vi "Drive_Notifier_Begin.vi"   [LabVIEW 2020]
uses:
  Subsystems/Drive/Drive_Cluster.ctl
  Subsystems/Drive/Drive_Control_States.ctl
  Subsystems/Drive/Drive_Orientation_States.ctl
  Globals/Drive_Globals.vi
types:
  T1 = typedef "Drive_Cluster.ctl" = cluster{"Control_State":T2, "Vertical_Throttle":dbl, "Lateral_Throttle":dbl, "Rotational_Throttle":dbl, "Strafe_In_Deadband":bool, "Rotation_In_Deadband":bool, "Orientation_State":T3, "Parameters":dbl[], "Step":i32, "Auto_Notifier":refnum<notifier>, "PathName":string, "Raw_X":dbl, "Raw_Y":dbl, "Pivot_Driving?":bool}
  T2 = typedef "Drive_Control_States.ctl" = enum16{"No-Op", "Manual_Control", "Command_DriveDistanceAtAngle", "Command_DrivePath", "Command_SetRobotPose", "Command_Rotate"}
  T3 = typedef "Drive_Orientation_States.ctl" = enum16{"Robot-Oriented", "Field-Oriented"}
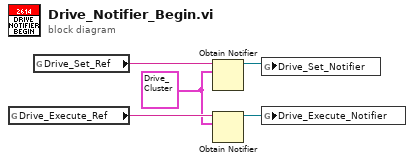
[diagram p0: block diagram]
diagram:
  w1 = T1 {"Control_State"=enum."No-Op", "Vertical_Throttle"=0.0, "Lateral_Throttle"=0.0, "Rotational_Throttle"=0.0, "Strafe_In_Deadband"=FALSE, "Rotation_In_Deadband"=FALSE, "Orientation_State"=enum."Robot-Oriented", "Parameters"=[], "Step"=0, "Auto_Notifier"=refnum, "PathName"="", "Raw_X"=0.0, "Raw_Y"=0.0, "Pivot_Driving?"=FALSE} ("Cluster")
  n1 = global read "Drive_Globals.vi" "Drive_Execute_Ref"() -> (w4:string)
  n2 = global read "Drive_Globals.vi" "Drive_Set_Ref"() -> (w5:string)
  n3 = Obtain Notifier(name (unnamed)=w5, notification data type=w1) -> (notifier out=w3:refnum<notifier>)  [unwired: 2 in, 2 out]
  n4 = Obtain Notifier(name (unnamed)=w4, notification data type=w1) -> (notifier out=w2:refnum<notifier>)  [unwired: 2 in, 2 out]
  n5 = global write "Drive_Globals.vi" "Drive_Set_Notifier"(w3) -> ()
  n6 = global write "Drive_Globals.vi" "Drive_Execute_Notifier"(w2) -> ()
